vi "CSM-FileSync.vi"(5 "Name(FileSync)":string="FileSync", 7 "Protocol.lvclass":refnum<class "Protocol.lvclass">, 8 "error in":errorcluster, 11 "FileSync Configuration":T1={"MonitoringFolder"=path "_sync/Monitoring", "BackupFolder"=path "_sync/backup", "autostart"=TRUE, "Backup"=FALSE}) -> (0 "error out":errorcluster)   [LabVIEW 2020, in "CSM-FileSync.lvlib"]
doc: "------------- lvcsm -------------\n[CSMStates]\nItem 0 = \"Idle\"\nItem 1 = \"Timeout\"\nItem 2 = \"Initialize Core Data\"\nItem 3 = \"Error Handler\"\nItem 4 = \"VI Reference\"\nItem 5 = \"Exit\"\nItem 6 = \"Data: Initialize\"\nItem 7 = \"Data: Load Configuration\"\nItem 8 = \"Data: Save Configuration\"\nItem 9 = \"Data: Cleanup\"\nItem 10 = \"UI: Initialize\"\nItem 11 = \"UI: Cursor Set\"\nItem 12 = \"UI: Front Panel State\"\nItem 13 = \"UI: Publish Status\"\nItem 14 = \"Macro: Initialize\"\nItem 15 = \"Macro: FileSync Protocol Connect\"\nItem 16 = \"Macro: Check Is Still Alive\"\nItem 17 = \"Macro: FileSync Routines\"\nItem 18 = \"Macro: FileSync Protocol Disconnect\"\nItem 19 = \"Macro: Exit\"\nItem 20 = \"API: Start\"\nItem 21 = \"API: Stop\"\nItem 22 = \"FileSync: Load Configuration\"\nItem 23 = \"FileSync: Try to Connect\"\nItem 24 = \"FileSync: Status Check\"\nItem 25 = \"FileSync: Close Connection\"\nItem 26 = \"FileSync: Cleanup Protocol\"\nItem 27 = \"FileSyncRountine: Create Dir if Not Exist\"\nItem 28 = \"FileSyncRountine: List Files\"\nItem 29 = \"FileSyncRountine: Pick Uploading File\"\nItem 30 = \"FileSyncRountine: Upload\"\nItem 31 = \"FileSyncRountine: Move File to Backup Folder\"\nItem 32 = \"FileSyncRountine: Remove Empty Container Folder\"\n\n[CSMStatus]\nItem 0 = \"Status Change@UI: Publish Status\"\nItem 1 = \"Uploading List Change@UI: Publish Status\""
uses:
  CSM-FileSync.lvlib
  _fileSync_Support/Base/Protocol/Protocol.lvclass
  _fileSync_Support/Base/Def-FileSyncConfig.ctl
  c11ad69d-c218-40bd-9883-d3361c9d07ec.vi
  4f3a877e-8c3a-40cf-89f4-fda6eeae6ffa.vi
  d714c97a-ade9-4c5a-b010-05319b638c8a.vi
  16b40464-5854-4f01-88e3-2a837e9228b3.vi
  16b40464-5854-4f01-88e3-2a837e9228b3.vi/eb2405bd-5b2e-436b-9bb3-692ecf4a9268.vi
  16b40464-5854-4f01-88e3-2a837e9228b3.vi/c8ad12e3-5e6d-40e1-92e0-1426ef45ec41.vi
  16b40464-5854-4f01-88e3-2a837e9228b3.vi/effcbc1a-e97c-42d4-b61f-d821de102707.vi
  <userlib>/_NEVSTOP/Communicable State Machine(CSM)/addons/MassData-Parameter/_support/FGV-MassData(lvlibp).vi
  <userlib>/_NEVSTOP/Communicable State Machine(CSM)/_Polymophic/Add State(s) to Queue By BOOL(Element).vi
  <userlib>/_NEVSTOP/Communicable State Machine(CSM)/_Polymophic/Build Status Broadcast Message.vi
  <userlib>/_NEVSTOP/Communicable State Machine(CSM)/AdvanceAPI/CSM - Set Module Attribute.vi
  <userlib>/_NEVSTOP/Communicable State Machine(CSM)/addons/API-String-Arugments-Support/_Support/Data To API String Arguments.vi
  <userlib>/_NEVSTOP/Communicable State Machine(CSM)/Communicable State Machine.lvlib
  <userlib>/_NEVSTOP/Communicable State Machine(CSM)/addons/Logger/CSM File Logger.lvlib
  <userlib>/_NEVSTOP/Communicable State Machine(CSM)/addons/Loop-Support/CSM Loop Support.lvlib
  <userlib>/_NEVSTOP/Communicable State Machine(CSM)/addons/MassData-Parameter/CSM MassData Parameter Support.lvlib
panel:
  out "State History":string
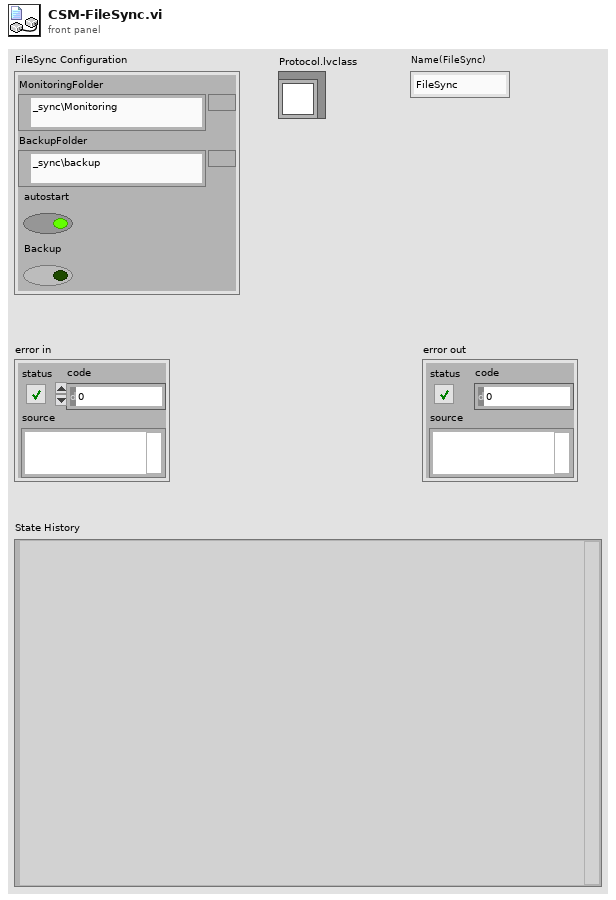
[diagram p1: front panel]
types:
  T1 = typedef "FileSync -- Base.lvlib/Protocol.lvclass/Def-FileSyncConfig.ctl" = cluster{"MonitoringFolder":path, "BackupFolder":path, "autostart":bool, "Backup":bool}
  T2 = enum32{"Invalid", "Standard", "Closed", "Hidden", "Minimized", "Maximized"}
  T3 = enum32{"invalid app kind", "Development System", "Run Time System", "Student Edition", "Embedded LabVIEW", "Evaluation", "Custom"}
  T4 = cluster{"Upload List":path[], "UploadingFile":path}
  T5 = typedef "Communicable State Machine.lvlib/_CSM_Response Source Message.ctl" = cluster{"‘State":string, "’Arguments":string, "’Error":errorcluster}
  T6 = cluster{"Core":cluster{"Current VI Reference":refnum<vi>, "Close Panel on Exit?":bool}, "Configuration":T1, "FileSync Status":cluster{"Connected":bool}, "Upload List":path[], "Temp:UploadingFile":path}
  T7 = cluster{"Current VI Reference":refnum<vi>, "Close Panel on Exit?":bool}
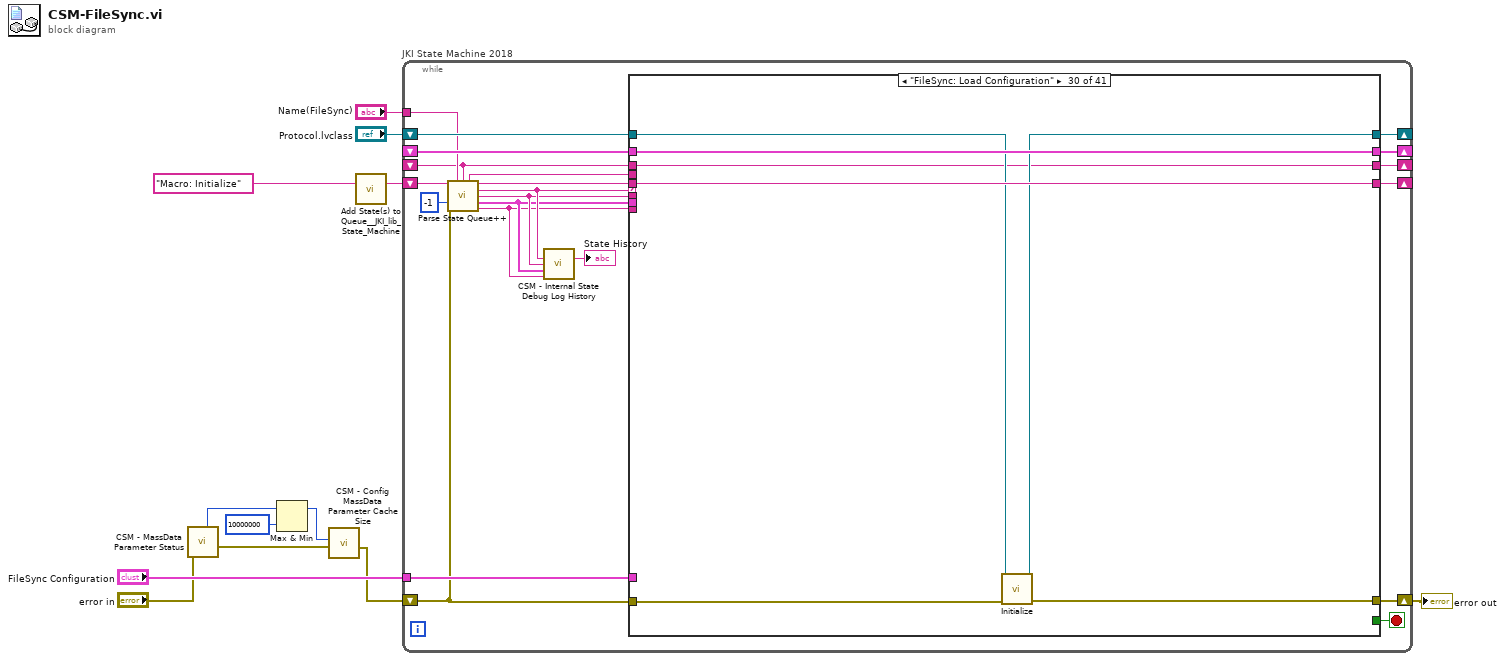
[diagram p0: block diagram]
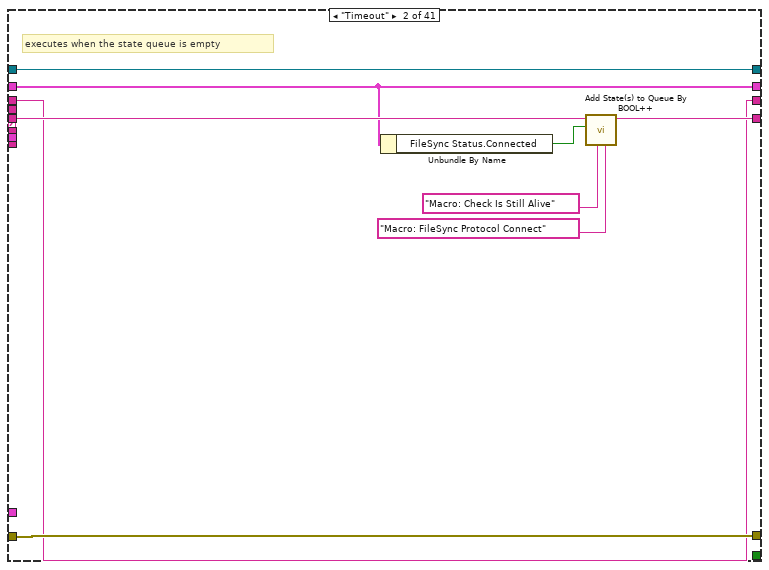
[diagram p3: hidden frame]
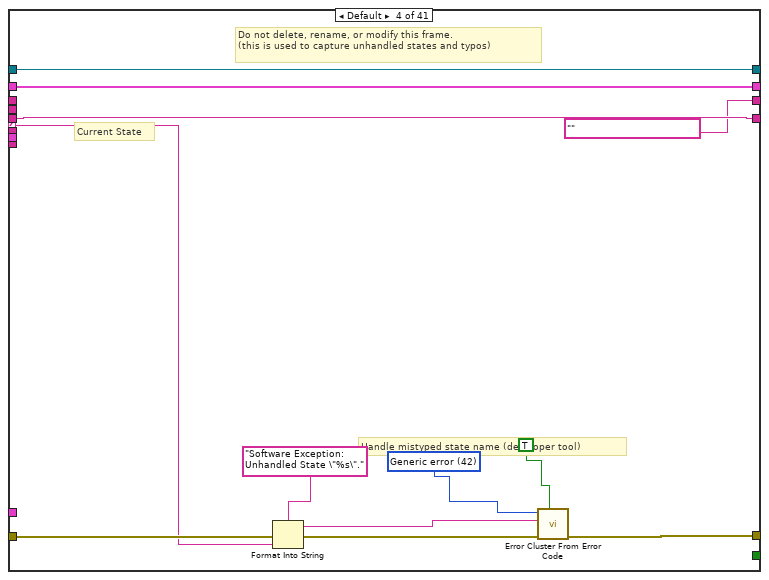
[diagram p5: hidden frame]
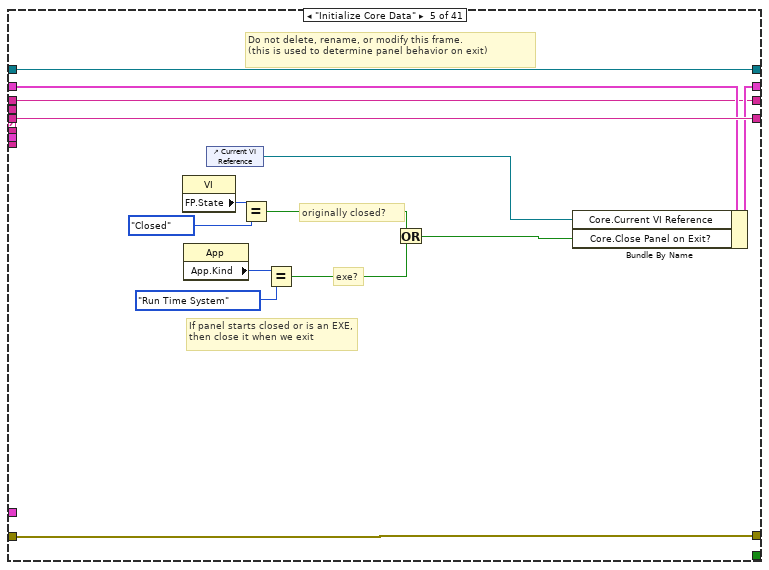
[diagram p6: hidden frame]
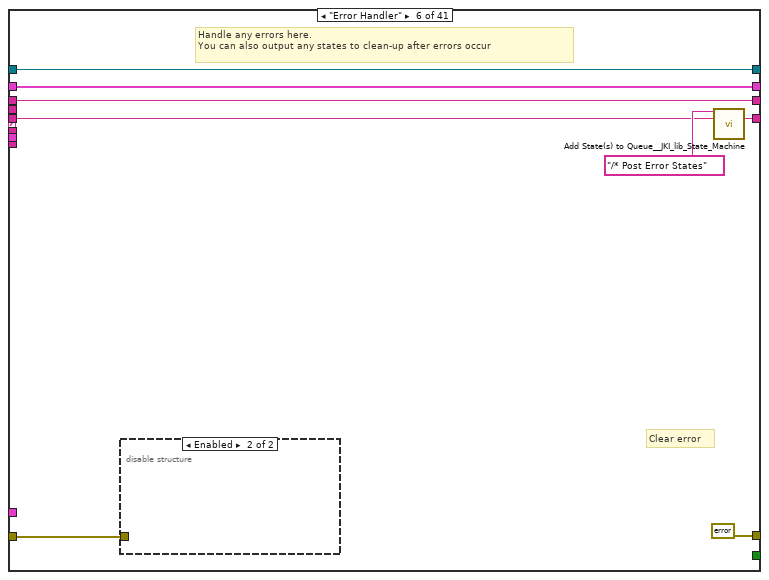
[diagram p7: hidden frame]
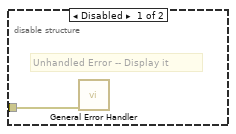
[diagram p8: hidden frame]
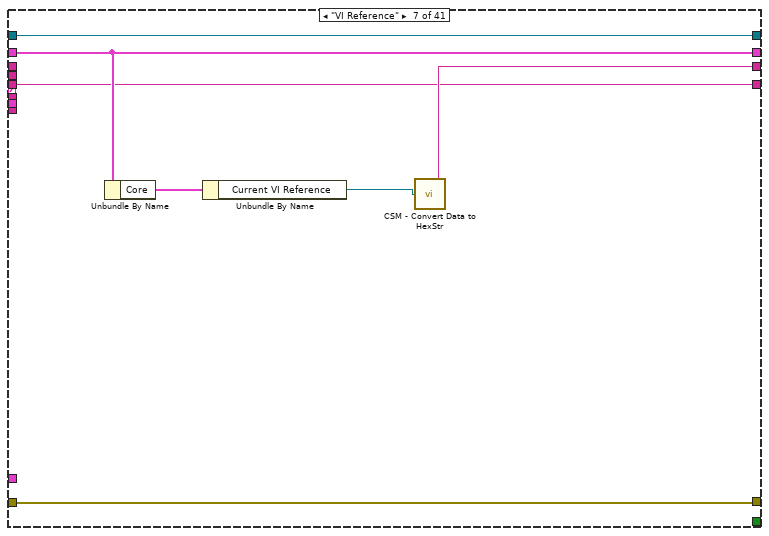
[diagram p9: hidden frame]
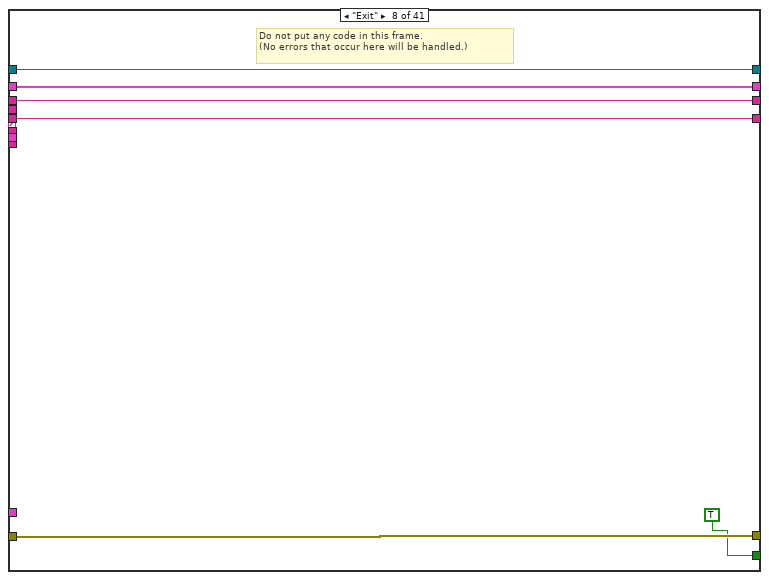
[diagram p10: hidden frame]
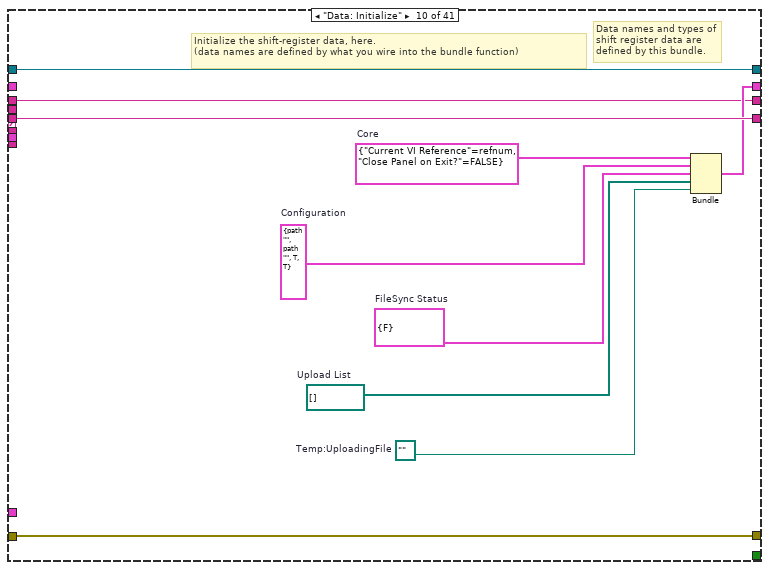
[diagram p12: hidden frame]
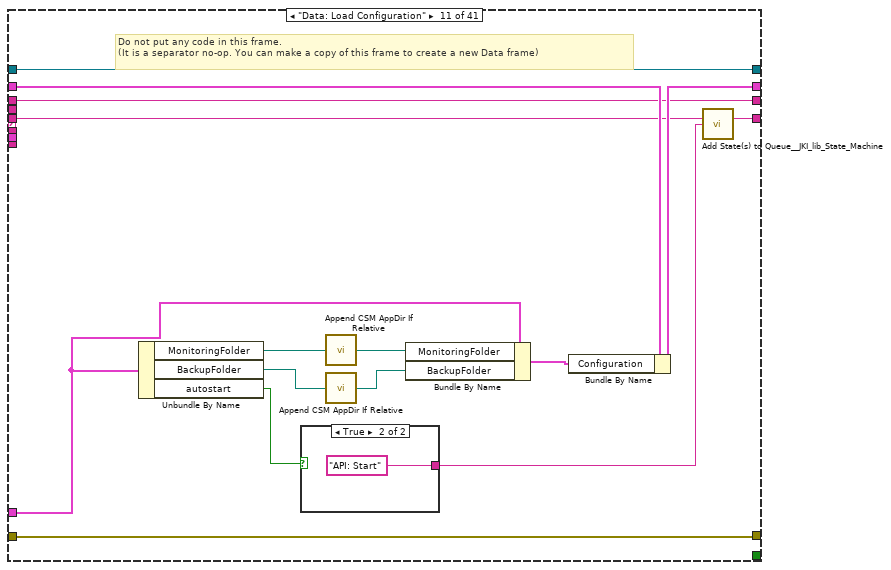
[diagram p13: hidden frame]
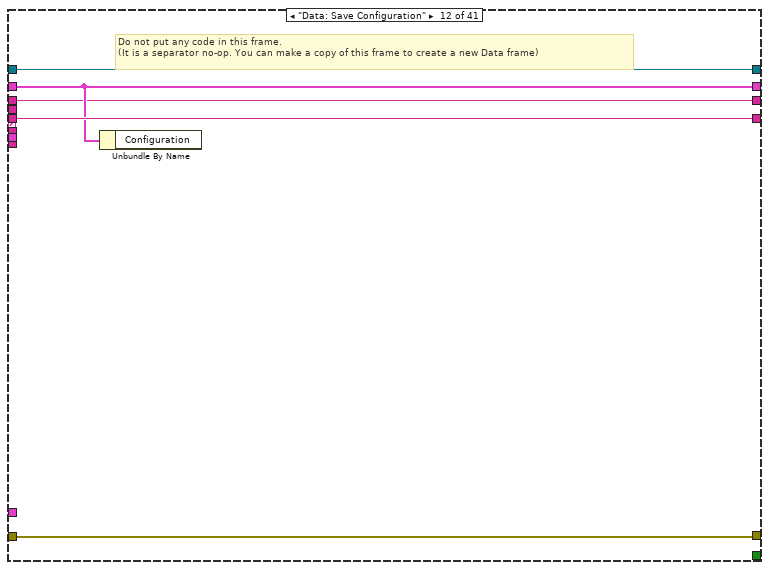
[diagram p15: hidden frame]
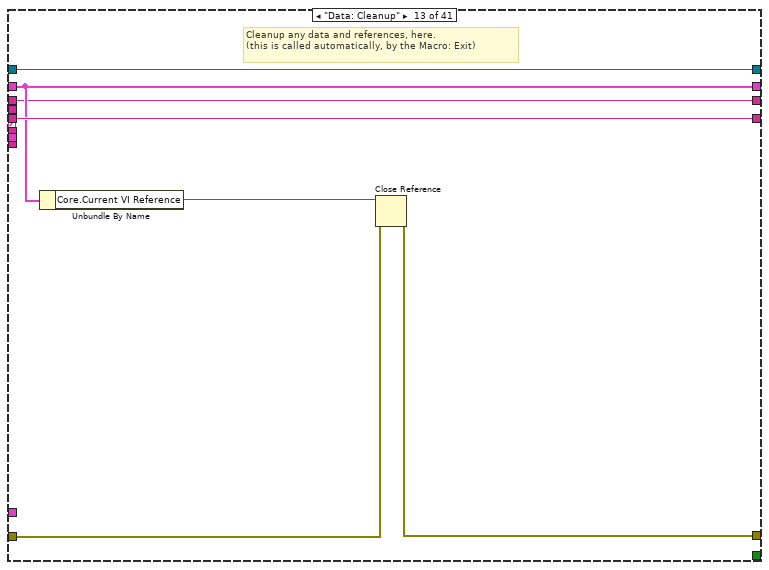
[diagram p16: hidden frame]
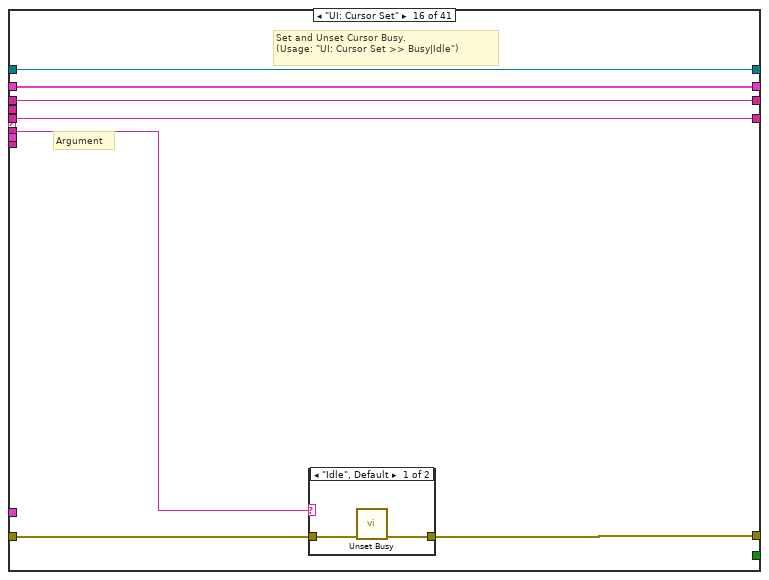
[diagram p19: hidden frame]
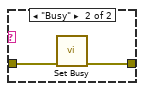
[diagram p20: hidden frame]
diagram:
  n1 = call <userlib>:"CSM - MassData Parameter Status.vi"("Error in"="error in") -> ("Error out"=w6:errorcluster, "Cache Size"=w2:i32)  [unwired: 6 in, 2 out]
  n2 = Max & Min(x=w2, y=10000000) -> (max(x,y)=w3:i32)  [unwired: 1 out]
  n3 = call <userlib>:"CSM - Config MassData Parameter Cache Size.vi"("Error in"=w6, "Size (50M)"=w3) -> ("Error out"=w5:errorcluster)  [unwired: 9 in]
  n4 = call <vilib>:"Add State(s) to Queue__JKI_lib_State_Machine.vi"("State(s) in (\"\")"="Macro: Initialize") -> ("States Out"=w12:string)  [unwired: 14 in]
  n5 = while "JKI State Machine 2018" {
    shift-right: [w30] -> _
    shift-left: _ -> [w29]
    shift-right: [w33] -> w10
    shift-left: w5 -> [w24]
    shift-right: [w32] -> _
    shift-left: w12 -> [w25]
    shift-right: [w27] -> _
    shift-left: "Protocol.lvclass" -> [w28]
    tunnel: "FileSync Configuration" -> [w26]
    shift-right: [w22] -> _
    shift-left: _ -> [w19]
    tunnel: "Name(FileSync)" -> [w21]
    stop <- w31 stop-if-true
    n6 = call <userlib>:"Parse State Queue++.vi"("State Queue"=w25, "Name (\"\" to Use UUID)"=w21, "Response Arguments"=w19, "Previous Error"=w24, "Dequeue (1 ms)"=-1 ("Dequeue Timeout(1ms)")) -> ("Name Used"=w20:string, "Remaining States"=w23:string, "Current State"=w17:string, "Arguments"=w16:string, "Additional Information"=w15:T5, "Source CSM"=w14:string)  [unwired: 5 in]
    n7 = call <userlib>:"CSM - Internal State Debug Log History.vi"("State"=w17, "Arguments (\"\")"=w16, ">> Response Source Message >>"=w15, "Source (\"\")"=w14) -> ("Debug Log"=→"State History":string)  [unwired: 11 in]
    n8 = case shown="\"FileSync: Load Configuration\"" w17 {
      selector: w17 -> [_ _ _ w55 _ _ _ _ _ _ _ _ _ _ _ _ _ _ _ _ _ _ _ _ _ _ _ _ _ _ _ w359 _ _ _ _ _ _ _ _ _]
      tunnel: w23 -> [w34 w47 w52 w58 w78 w79 w90 w100 w105 w115 w119 w136 w143 w148 w153 w160 w172 w250 w262 w269 w274 w282 w293 w302 w318 w321 w327 w332 w338 w345 w354 w360 w377 w384 w389 w397 w406 w422 w432 w458 w500]
      tunnel: w16 -> [_ _ _ _ _ _ _ _ _ _ _ _ _ _ _ w156 w167 _ _ _ _ _ _ _ _ _ _ _ _ _ _ _ _ _ _ _ _ _ w440 w449 w494]
      tunnel: w29 -> [w37 w44 w50 w57 w72 w84 w94 w99 w103 _ w128 w134 w139 w146 w152 w159 w169 w255 w260 w266 w272 w280 w291 w300 w315 w320 w326 w331 w336 w344 w353 w364 w376 w383 w387 w394 w404 w418 w437 w456 w496]
      tunnel: [w38 w45 w51 w60 w76 errorcluster {"status"=FALSE, "code"=0, "source"=""} ("error out") w89 w98 w104 w113 w127 w133 w140 w147 w151 w157 w170 w256 w261 w267 w276 w284 w295 w304 w316 w322 w328 w333 w337 w342 w349 w367 w374 w381 w388 w390 w402 w420 w424 w453 w497] -> w33
      tunnel: w24 -> [w38 w45 w51 w59 w76 w83 w89 w98 w104 w113 w127 w133 w141 w147 w151 w158 w171 w256 w261 w267 w276 w284 w295 w304 w316 w322 w328 w333 w337 w343 w350 w368 w375 w382 w388 _ w401 w420 w438 _ w498]
      tunnel: [w34 w46 w52 w58 w78 w86 w90 w100 w105 w115 w120 w136 w143 w148 w153 w160 w172 w251 w262 w268 w275 w283 w294 w303 w317 w321 w324 w329 w338 w345 w354 w361 w377 w384 w389 w397 w406 w421 w433 w458 w500] -> w32
      tunnel: [_ _ _ _ _ _ _ TRUE _ _ _ _ _ _ _ _ _ _ _ _ _ _ _ _ _ _ _ _ _ _ _ _ _ _ _ _ _ _ _ _ _] -> w31
      tunnel: [w37 w44 w50 w57 w77 w84 w94 w99 w103 w114 w129 w134 w139 w146 w152 w159 w169 w255 w260 w266 w272 w280 w291 w300 w315 w320 w326 w331 w336 w344 w348 w364 w371 w383 w387 w394 w400 w417 w437 w450 w496] -> w30
      tunnel: w28 -> [w36 w43 w49 w54 w66 w81 w88 w96 w102 w111 w130 w135 w138 w145 w150 w155 w166 w257 w259 w264 w277 w285 w296 w305 w308 w319 w325 w330 w335 w341 w352 w366 w373 w380 w386 w396 w405 w419 w435 w457 w499]
      tunnel: [w36 w43 w49 w54 w66 w81 w88 w96 w102 w111 w130 w135 w138 w145 w150 w155 w166 w257 w259 w264 w277 w285 w296 w305 w308 w319 w325 w330 w335 w340 w351 w365 w372 w379 w386 w396 w405 w419 w439 w457 w499] -> w27
      tunnel: w26 -> [_ _ _ _ _ _ _ _ _ _ w116 _ _ _ _ _ _ _ _ _ _ _ _ _ _ _ _ _ _ _ _ _ _ _ _ _ _ _ _ _ _]
      tunnel: [w35 w42 w48 "" ("message") w65 w80 w91 w95 w101 w106 w125 w132 w137 w144 w149 w154 w165 w254 w258 w263 w270 w279 w292 w298 w307 _ _ _ w334 w339 w346 w363 w369 w378 w385 w391 w398 w410 w434 w452 w491] -> w22
      tunnel: w14 -> [_ _ _ _ _ _ _ _ _ _ _ _ _ _ _ _ _ _ _ _ _ _ _ _ _ _ _ _ _ _ _ _ _ _ _ _ _ _ _ _ _]
      tunnel: w15 -> [_ _ _ _ _ _ _ _ _ _ _ _ _ _ _ _ _ _ _ _ _ _ _ _ _ _ _ _ _ _ _ _ _ _ _ _ _ _ _ _ _]
      tunnel: w20 -> [_ _ _ _ _ _ _ _ _ _ _ _ _ _ _ _ _ w253 _ _ _ _ _ _ _ _ _ _ _ _ _ _ _ _ _ _ _ _ _ _ _]
      tunnel: w19 -> [w35 w42 w48 _ w65 w80 _ w95 w101 w106 w125 w132 w137 w144 w149 w154 w165 w254 w258 w263 w270 w279 w292 w298 w307 _ _ _ w334 w339 w346 w363 w369 w378 w385 w391 w398 w410 w434 w452 w491]
      frame "", "Idle" {
      }
      frame "Timeout" {
        # "executes when the state queue is empty"
        n9 = Unbundle By Name(w44) -> ("FileSync Status.Connected"=w39:bool)
        n10 = call-poly <userlib>:"Add State(s) to Queue By BOOL++.vi"("FALSE (\"\")"="Macro: FileSync Protocol Connect" ("State(s) in Front (\"\")"), "TRUE (\"\")"="Macro: Check Is Still Alive" ("State(s) in Front (\"\")"), "Condition"=w39, "State Queue (\"\")"=w47) -> ("Remaining States"=w46:string)  [unwired: 7 in]
      }
      frame "---------- Core ----------" {
        # "Do not put any code in this frame.\n(it is a separator no-op)"
      }
      frame Default {
        w63 = 42 items=["No error", "Argument error", "Memory is full", "Out of zone", "End of file", "File already open", "Generic file I/O error", "File not found", "File permission error", "Disk is full", "Duplicate path", "Too many files open", "System feature not enabled", "Resource file not found", "Cannot add resource", "Resource not found", "Image not found", "Image memory error", "Pen does not exist", "Config type invalid", "Config token not found", "Config parse error", "Config memory error", "Bad external code format", "Bad external code offset", "External code not present", "Null window", "Destroy window error", "Null menu", "Print aborted", "Bad print record", "Print driver error", "Windows error during printing", "Memory error during printing", "Print dialog error", "Generic print error", "Invalid device refnum", "Device not found", "Device parameter error", "Device unit error", "Cannot open device", "Device call aborted", "Generic error", "Cancelled by user", "Object ID too low", "Object ID too high", "Object not in heap", "Unknown heap", "Unknown object (invalid DefProc)", "Unknown object (DefProc not in table)", "Message out of range", "Invalid (null) method", "Unknown message", "Manager call not supported", "Bad address", "Network operation in progress", "Network operation timed out", "Connection is busy", "Network attribute not supported", "Network error", "Address in use", "System out of memory", "Connection aborted", "Connection refused", "Not connected", "Already connected", "Connection closed", "Initialization error (interapplication manager)", "Bad occurrence", "Wait on unbound occurrence handler", "Occurrence queue overflow", "Datalog type conflict", "Unused", "Unrecognized type (interapplication manager)", "Memory corrupt", "Failed to make temporary DLL", "Old CIN version", "Drag socket not found", "Failed to load drop-object", "Failed to register OLE object", "Failed to release OLE object", "Format specifier type mismatch", "Unknown format specifier", "Too few format specifiers", "Too many format specifiers", "Scan failed", "Newer CIN version", "Error converting to variant", "Runtime menu error", "Password tampered", "Variant attribute not found", "Incompatible variant data type", "Event data is not available", "Event Store is not present", "Occurrence is not found", "Event Queue is not created", "Event info is not available", "Refnum passed is NULL", "Error retrieving Class GUID", "Error retrieving CoClass GUID", "Error retrieving TypeLib GUID.", "Bad built application magic bytes.", "Specific driver is different from the specific driver associated with the Logical Name.", "There is no session opened to the class driver.", "Max Error", "MAX - Error with config objects", "MAX - Error loading configuration", "MAX - Group not supported"]
        # "Current State"
        # "Do not delete, rename, or modify this frame.\n(this is used to capture unhandled states and typos)"
        # "Handle mistyped state name (developer tool)"
        n11 = Format Into String(format string="Software Exception: Unhandled State \"%s\"." ("message"), error in=w59, w55) -> (resulting string=w62:string, error out=w61:errorcluster)  [unwired: 1 in]
        n12 = call <vilib>:"Error Cluster From Error Code.vi"("show call chain? (False)"=TRUE, "error in (no error)"=w61, "error message (\"\")"=w62, "error code (0)"=w63) -> ("error out"=w60:errorcluster)  [unwired: 5 in]
      }
      frame "Initialize Core Data" {
        # "Do not delete, rename, or modify this frame.\n(this is used to determine panel behavior on exit)"
        # "originally closed?"
        # "exe?"
        # "If panel starts closed or is an EXE, then close it when we exit"
        n13 = property class="VI"() -> ("FP.State"=w69:T2)  [unwired: 2 in, 2 out]
        n14 = property class="App"() -> ("App.Kind"=w75:T3)  [unwired: 2 in, 2 out]
        n15 = control-ref of="Current VI Reference"() -> (w70:refnum<vi>)
        n16 = Equal?(x=w69, y=T2."Closed" ("Front Panel Window:State")) -> (x = y?=w67:bool)
        n17 = Equal?(x=w75, y=T3."Run Time System" ("Application:Kind")) -> (x = y?=w73:bool)
        n18 = Or(x=w67, y=w73) -> (x .or. y?=w71:bool)
        n19 = Bundle By Name(cluster=w72, "Core.Current VI Reference"=w70, "Core.Close Panel on Exit?"=w71) -> (w77:T6)
      }
      frame "Error Handler" {
        # "Handle any errors here.\nYou can also output any states to clean-up after errors occur"
        # "Clear error"
        n20 = disable-structure shown="Enabled" {
          disable-tunnel: w83 -> [w87 _]
          frame Disabled {
            # "Unhandled Error -- Display it"
            n21 = call <vilib>:"General Error Handler.vi"("error in (no error)"=w87) -> ()  [unwired: 10 in, 5 out]
          }
          frame Enabled {
          }
        }
        n22 = call <vilib>:"Add State(s) to Queue__JKI_lib_State_Machine.vi"("State(s) in Front (\"\")"="/* Post Error States", "State(s) in (\"\")"=w79) -> ("States Out"=w86:string)  [unwired: 13 in]
      }
      frame "VI Reference" {
        n23 = Unbundle By Name(w94) -> ("Core"=w93:T7)
        n24 = Unbundle By Name(w93) -> ("Current VI Reference"=w92:refnum<vi>)
        n25 = call <userlib>:"CSM - Convert Data to HexStr.vi"("Variant"=w92) -> ("HEX String (0-9,A-F)"=w91:string)  [unwired: 8 in]
      }
      frame "Exit" {
        # "Do not put any code in this frame.\n(No errors that occur here will be handled.)"
      }
      frame "---------- Data ----------" {
        # "Do not put any code in this frame.\n(It is a separator no-op. You can make a copy of this frame to create a new Data frame)"
      }
      frame "Data: Initialize" {
        w107 = path ""  # Temp:UploadingFile
        w108 = path[] []  # Upload List
        w109 = cluster{"Connected":bool} {"Connected"=FALSE}  # FileSync Status
        w110 = T1 {"MonitoringFolder"=path "", "BackupFolder"=path "", "autostart"=TRUE, "Backup"=TRUE}  # Configuration
        w112 = T7 {"Current VI Reference"=refnum, "Close Panel on Exit?"=FALSE}  # Core
        # "Data names and types of shift register data are defined by this bundle."
        # "Initialize the shift-register data, here.\n(data names are defined by what you wire into the bundle function)"
        n26 = Bundle("Core"=w112, "Configuration"=w110, "FileSync Status"=w109, "Upload List"=w108, "Temp:UploadingFile"=w107) -> (w114:T6)  [unwired: 1 in]
      }
      frame "Data: Load Configuration" {
        # "Do not put any code in this frame.\n(It is a separator no-op. You can make a copy of this frame to create a new Data frame)"
        n27 = Unbundle By Name(w116) -> ("MonitoringFolder"=w124:path, "BackupFolder"=w123:path, "autostart"=w117:bool)
        n28 = case shown="True" w117 {
          tunnel: [_ "API: Start" ("State(s) at Back (\"\")")] -> w118
          frame False {
          }
          frame True {
          }
        }
        n29 = call <userlib>:"Append CSM AppDir If Relative.vi"("Relative Path (.)"=w124) -> ("Application Directory (+ Relative)"=w122:path)  [unwired: 4 in]
        n30 = call <userlib>:"Append CSM AppDir If Relative.vi"("Relative Path (.)"=w123) -> ("Application Directory (+ Relative)"=w121:path)  [unwired: 4 in]
        n31 = Bundle By Name(cluster=w116, "MonitoringFolder"=w122, "BackupFolder"=w121) -> (w126:T1)
        n32 = Bundle By Name(cluster=w128, "Configuration"=w126) -> (w129:T6)
        n33 = call <vilib>:"Add State(s) to Queue__JKI_lib_State_Machine.vi"("State(s) in (\"\")"=w119, "State(s) at Back (\"\")"=w118) -> ("States Out"=w120:string)  [unwired: 13 in]
      }
      frame "Data: Save Configuration" {
        # "Do not put any code in this frame.\n(It is a separator no-op. You can make a copy of this frame to create a new Data frame)"
        n34 = Unbundle By Name(w134) -> ()  [unwired: 1 out]
      }
      frame "Data: Cleanup" {
        # "Cleanup any data and references, here.\n(this is called automatically, by the Macro: Exit)"
        n35 = Unbundle By Name(w139) -> ("Core.Current VI Reference"=w142:refnum<vi>)
        n36 = Close Reference(reference=w142, error in (no error)=w141) -> (error out=w140:errorcluster)
      }
      frame "---------- UI ----------" {
        # "Do not put any code in this frame.\n(It is a separator no-op. You can make a copy of this frame to create a new UI frame)"
      }
      frame "UI: Initialize" {
      }
      frame "UI: Cursor Set" {
        # "Argument"
        # "Set and Unset Cursor Busy.\n(Usage: \"UI: Cursor Set >> Busy|Idle\")"
        n37 = case shown="\"Idle\", Default" w156 {
          tunnel: w158 -> [w162 w164]
          tunnel: [w161 w163] -> w157
          frame "Idle", Default {
            n38 = call <vilib>:"Unset Busy.vi"("error in (no error)"=w162) -> ("error out"=w161:errorcluster)  [unwired: 10 in]
          }
          frame "Busy" {
            n39 = call <vilib>:"Set Busy.vi"("error in (no error)"=w164) -> ("error out"=w163:errorcluster)  [unwired: 9 in, 1 out]
          }
        }
      }
      frame "UI: Front Panel State" {
        # "Argument"
        # "Set Front Panel Open or Closed\n(Usage: \"UI: Front Panel State >> Open|Close\")"
        n40 = Unbundle By Name(w169) -> ("Core.Current VI Reference"=w168:refnum<vi>)
        n41 = case shown="\"Open\", \"Standard\", Default" w167 {
          tunnel: w171 -> [w178 w193 w204 w217 w230]
          tunnel: [w180 w194 w206 w219 w232] -> w170
          tunnel: w168 -> [w179 w191 w205 w218 w231]
          frame "Open", "Standard", Default {
            w173 = T2."Standard" ("State")
            n42 = property class="VI"(reference=w179, error in=w178) -> (reference out=w176:refnum<vi>, error out=w177:errorcluster, "FP.State"=w175:T2)
            n43 = Not Equal?(x=w175, y=w173) -> (x != y?=w174:bool)
            n44 = case shown="True" w174 {
              tunnel: [w184 w186] -> w180
              tunnel: w177 -> [w183 w186]
              tunnel: w176 -> [w182 _]
              tunnel: w173 -> [w181 _]
              frame True {
                n45 = invoke class="VI" method="FP.Open"(reference=w182, error in=w183, "Activate"=TRUE, "State"=w181) -> (error out=w184:errorcluster)  [unwired: 1 in, 4 out]
              }
              frame False {
              }
            }
          }
          frame "Close", "Closed" {
            n46 = property class="VI"(reference=w191, error in=w193) -> (reference out=w190:refnum<vi>, error out=w192:errorcluster, "FP.State"=w188:T2)
            n47 = Not Equal?(x=w188, y=T2."Closed" ("Front Panel Window:State")) -> (x != y?=w187:bool)
            n48 = case shown="True" w187 {
              tunnel: [w195 w198] -> w194
              tunnel: w192 -> [w195 w197]
              tunnel: w190 -> [_ w196]
              frame False {
              }
              frame True {
                n49 = invoke class="VI" method="FP.Close"(reference=w196, error in=w197) -> (error out=w198:errorcluster)  [unwired: 1 in, 2 out]
              }
            }
          }
          frame "Hidden", "Hide" {
            w199 = T2."Hidden" ("State")
            n50 = property class="VI"(reference=w205, error in=w204) -> (reference out=w202:refnum<vi>, error out=w203:errorcluster, "FP.State"=w201:T2)
            n51 = Not Equal?(x=w201, y=w199) -> (x != y?=w200:bool)
            n52 = case shown="True" w200 {
              tunnel: [w210 w211] -> w206
              tunnel: w203 -> [w209 w211]
              tunnel: w202 -> [w208 _]
              tunnel: w199 -> [w207 _]
              frame True {
                n53 = invoke class="VI" method="FP.Open"(reference=w208, error in=w209, "State"=w207) -> (error out=w210:errorcluster)  [unwired: 2 in, 4 out]
              }
              frame False {
              }
            }
          }
          frame "Minimize", "Minimized" {
            w212 = T2."Minimized" ("State")
            n54 = property class="VI"(reference=w218, error in=w217) -> (reference out=w215:refnum<vi>, error out=w216:errorcluster, "FP.State"=w214:T2)
            n55 = Not Equal?(x=w214, y=w212) -> (x != y?=w213:bool)
            n56 = case shown="True" w213 {
              tunnel: [w223 w224] -> w219
              tunnel: w216 -> [w222 w224]
              tunnel: w215 -> [w221 _]
              tunnel: w212 -> [w220 _]
              frame True {
                n57 = invoke class="VI" method="FP.Open"(reference=w221, error in=w222, "State"=w220) -> (error out=w223:errorcluster)  [unwired: 2 in, 4 out]
              }
              frame False {
              }
            }
          }
          frame "Maximize", "Maximized" {
            w225 = T2."Maximized" ("State")
            n58 = property class="VI"(reference=w231, error in=w230) -> (reference out=w228:refnum<vi>, error out=w229:errorcluster, "FP.State"=w227:T2)
            n59 = Not Equal?(x=w227, y=w225) -> (x != y?=w226:bool)
            n60 = case shown="True" w226 {
              tunnel: [w236 w237] -> w232
              tunnel: w229 -> [w235 w237]
              tunnel: w228 -> [w234 _]
              tunnel: w225 -> [w233 _]
              frame True {
                n61 = invoke class="VI" method="FP.Open"(reference=w234, error in=w235, "State"=w233) -> (error out=w236:errorcluster)  [unwired: 2 in, 4 out]
              }
              frame False {
              }
            }
          }
        }
      }
      frame "UI: Publish Status" {
        n62 = Unbundle By Name(w255) -> ("FileSync Status.Connected"=w249:bool, "Upload List"=w238:path[], "Temp:UploadingFile"=w248:path)
        n63 = call "CSM Set Module Attribute.vim"("CSM Name"=w253, "Attribute"="Connected", "Value"=w249) -> ()  [unwired: 9 in, 4 out]
        n64 = Bundle(cluster=T4 {"Upload List"=[], "UploadingFile"=path ""} ("output cluster"), "Upload List"=w238, "UploadingFile"=w248) -> (w246:T4)
        n65 = call "Convert Data To API String Arguments.vim"("Data"=w249) -> ("API String"=w239:string)  [unwired: 7 in, 1 out]
        n66 = call "CSM - Convert MassData to Argument.vim"("Data"=w246) -> ("MassData Argument"=w241:string)  [unwired: 7 in, 1 out]
        n67 = call-poly <userlib>:"Build Message with Arguments++.vi"("State With Arguments"="Status Change" ("Attribute"), "Arguments (\"\")"=w239) -> ("CSM Message String"=w245:string)  [unwired: 13 in]
        n68 = call-poly <userlib>:"Build Message with Arguments++.vi"("State With Arguments"="Uploading List Change" ("Attribute"), "Arguments (\"\")"=w241) -> ("CSM Message String"=w244:string)  [unwired: 13 in]
        n69 = call <vilib>:"Add State(s) to Queue__JKI_lib_State_Machine.vi"("State(s) in (\"\")"=w245, "State(s) at Back (\"\")"=w244) -> ("States Out"=w243:string)  [unwired: 13 in]
        n70 = call <vilib>:"Add State(s) to Queue__JKI_lib_State_Machine.vi"("State(s) in Front (\"\")"=w243, "State(s) in (\"\")"=w250) -> ("States Out"=w251:string)  [unwired: 13 in]
      }
      frame "---------- Macro ----------" {
        # "Do not put any code in this frame.\n(It is a separator no-op. You can make a copy of this frame to create a new Macro frame)"
      }
      frame "Macro: Initialize" {
        # "Initialization Macro\n(This is called once, when the VI starts)"
        n71 = call <vilib>:"Add State(s) to Queue__JKI_lib_State_Machine.vi"("State(s) in Front (\"\")"="Data: Initialize\nInitialize Core Data\nData: Load Configuration\nUI: Initialize\nUI: Publish Status\n//UI: Front Panel State >> Open\n", "State(s) in (\"\")"=w269) -> ("States Out"=w268:string)  [unwired: 13 in]
      }
      frame "Macro: FileSync Protocol Connect" {
        n72 = Unbundle By Name(w272) -> ("FileSync Status.Connected"=w271:bool)
        n73 = case shown="True" w271 {
          tunnel: [_ "FileSync: Load Configuration\nFileSync: Try to Connect\nUI: Publish Status" ("State(s) in Front (\"\")")] -> w273
          frame False {
          }
          frame True {
          }
        }
        n74 = call <vilib>:"Add State(s) to Queue__JKI_lib_State_Machine.vi"("State(s) in Front (\"\")"=w273, "State(s) in (\"\")"=w274) -> ("States Out"=w275:string)  [unwired: 13 in]
      }
      frame "Macro: Check Is Still Alive" {
        n75 = call <vilib>:"Add State(s) to Queue__JKI_lib_State_Machine.vi"("State(s) in Front (\"\")"="FileSync: Check Connection is Still Alive" ("State(s) in Front (\"\")"), "State(s) in (\"\")"=w282) -> ("States Out"=w283:string)  [unwired: 13 in]
      }
      frame "Macro: FileSync Routines" {
        n76 = Unbundle By Name(w291) -> ("Upload List"=w290:path[])
        n77 = Empty Array?(array=w290) -> (empty?=w286:bool)
        n78 = case shown="True" w286 {
          tunnel: [_ "FileSyncRountine: Create Dir if Not Exist\nFileSyncRountine: List Files" ("State(s) in Front (\"\")")] -> w289
          frame False {
          }
          frame True {
          }
        }
        n79 = call <vilib>:"Add State(s) to Queue__JKI_lib_State_Machine.vi"("State(s) in Front (\"\")"=w289, "State(s) in (\"\")"="FileSyncRountine: Pick Uploading File\n" ("State(s) in Front (\"\")")) -> ("States Out"=w287:string)  [unwired: 13 in]
        n80 = call <vilib>:"Add State(s) to Queue__JKI_lib_State_Machine.vi"("State(s) in Front (\"\")"=w287, "State(s) in (\"\")"=w293) -> ("States Out"=w294:string)  [unwired: 13 in]
      }
      frame "Macro: FileSync Protocol Disconnect" {
        n81 = Unbundle By Name(w300) -> ("FileSync Status.Connected"=w299:bool)
        n82 = case shown="True" w299 {
          tunnel: [_ "FileSync: Close Connection\nFileSync: Cleanup Protocol\nUI: Publish Status" ("State(s) in Front (\"\")")] -> w301
          frame False {
          }
          frame True {
          }
        }
        n83 = call <vilib>:"Add State(s) to Queue__JKI_lib_State_Machine.vi"("State(s) in Front (\"\")"=w301, "State(s) in (\"\")"=w302) -> ("States Out"=w303:string)  [unwired: 13 in]
      }
      frame "Macro: Exit" {
        # "Exit Macro\n(This is called once, when the VI exits)"
        n84 = Unbundle By Name(w315) -> ("Core.Close Panel on Exit?"=w314:bool)
        n85 = Select(t="//UI: Front Panel State >> Close", s=w314, f="") -> (s? t:f=w311:string)
        n86 = call <vilib>:"Add State(s) to Queue__JKI_lib_State_Machine.vi"("State(s) in (\"\")"=w311, "State(s) at Back (\"\")"="Macro: FileSync Protocol Disconnect\nData: Cleanup\nExit") -> ("States Out"=w309:string)  [unwired: 13 in]
        n87 = call <vilib>:"Add State(s) to Queue__JKI_lib_State_Machine.vi"("State(s) in Front (\"\")"=w309, "State(s) in (\"\")"=w318) -> ("States Out"=w317:string)  [unwired: 13 in]
      }
      frame "---------- API ----------" {
      }
      frame "API: Start" {
        n88 = call <userlib>:"CSMLS - Define Loop State(s).vi"("Loop States"="FileSync: Load Configuration\nFileSync: Try to Connect\nFileSync: Status Check -><loop>\nFileSync: Close Connection\nFileSync: Cleanup Protocol" ("Loop State(s) and Arguments"), "States Queue"=w327) -> ("Remaining States"=w324:string)  [unwired: 13 in]
      }
      frame "API: Stop" {
        n89 = call <userlib>:"CSMLS - Remove Loop Tag and previous State(s) to Break.vi"("States Queue"=w332) -> ("Remaining States"=w329:string)  [unwired: 10 in]
      }
      frame "---------- FileSync ----------" {
      }
      frame "FileSync: Load Configuration" {
        n90 = call-dynamic "Initialize.vi"("error in (no error)"=w343, "Protocol in"=w341) -> ("error out"=w342:errorcluster, "Protocol out"=w340:refnum<class "Protocol.lvclass">)  [unwired: 8 in]
      }
      frame "FileSync: Try to Connect" {
        n91 = call-dynamic "Connect.vi"("error in (no error)"=w350, "Protocol in"=w352) -> ("error out"=w349:errorcluster, "Connected?"=w347:bool, "Protocol out"=w351:refnum<class "Protocol.lvclass">)  [unwired: 7 in]
        n92 = Bundle By Name(cluster=w353, "FileSync Status.Connected"=w347) -> (w348:T6)
      }
      frame "FileSync: Status Check" {
        n93 = call-dynamic "Check.vi"("error in (no error)"=w368, "Protocol in"=w366) -> ("error out"=w367:errorcluster, "Still alive?"=w362:bool, "Protocol out"=w365:refnum<class "Protocol.lvclass">)  [unwired: 7 in]
        n94 = Wait (ms)(milliseconds to wait=u32 200) -> ()  [unwired: 1 out]
        n95 = Select(t="Macro: FileSync Routines" ("State(s) in Front (\"\")"), s=w362, f="Macro: FileSync Protocol Disconnect\nFileSync: Load Configuration\nFileSync: Try to Connect" ("State(s) in Front (\"\")")) -> (s? t:f=w357:string)
        n96 = call <userlib>:"CSMLS - Append Continuous State.vi"("Loop State(s) And Arguments"=w357, "Continous State"=w359, "States Queue"=w360) -> ("Remaining States"=w361:string)  [unwired: 8 in]
      }
      frame "FileSync: Close Connection" {
        n97 = call-dynamic "Disconnect.vi"("error in (no error)"=w375, "Protocol in"=w373) -> ("error out"=w374:errorcluster, "Protocol out"=w372:refnum<class "Protocol.lvclass">)  [unwired: 8 in]
        n98 = Bundle By Name(cluster=w376, "FileSync Status.Connected"=FALSE) -> (w371:T6)
      }
      frame "FileSync: Cleanup Protocol" {
        n99 = call-dynamic "Cleanup.vi"("error in (no error)"=w382, "Protocol in"=w380) -> ("error out"=w381:errorcluster, "Protocol out"=w379:refnum<class "Protocol.lvclass">)  [unwired: 8 in]
      }
      frame "---------- FileSyncRountine ----------" {
      }
      frame "FileSyncRountine: Create Dir if Not Exist" {
        n100 = Unbundle By Name(w394) -> ("Configuration.MonitoringFolder"=w393:path, "Configuration.BackupFolder"=w392:path)
        n101 = call <vilib>:"Create Directory Recursive.vi"("directory"=w393) -> ("error out"=w395:errorcluster)  [unwired: 4 in, 2 out]
        n102 = call <vilib>:"Create Directory Recursive.vi"("error in (no error)"=w395, "directory"=w392) -> ("error out"=w390:errorcluster)  [unwired: 3 in, 2 out]
      }
      frame "FileSyncRountine: List Files" {
        n103 = Unbundle By Name(w404) -> ("Configuration.MonitoringFolder"=w403:path)
        n104 = call <vilib>:"Recursive File List.vi"("error in (no error)"=w401, "Folder Path"=w403) -> ("error out"=w402:errorcluster, "All Files in Dir"=w399:path[])  [unwired: 5 in, 3 out]
        n105 = Bundle By Name(cluster=w404, "Upload List"=w399) -> (w400:T6)
      }
      frame "FileSyncRountine: Pick Uploading File" {
        n106 = Unbundle By Name(w418) -> ("Upload List"=w412:path[])
        n107 = Index Array(array=w412) -> (element=w411:path)  [unwired: 1 in]
        n108 = Path To String(path=w411) -> (string=w413:string)
        n109 = Bundle By Name(cluster=w418, "Temp:UploadingFile"=w411) -> (w417:T6)
        n110 = Empty String/Path?(string/path=w411) -> (empty?=w416:bool)
        n111 = call <vilib>:"Build State String with Arguments__JKI_lib_State_Machine.vi"("Arguments (\"\")"=w413, "State"="FileSyncRountine: Upload" ("False(Empty)")) -> ("State with Arguments"=w408:string)  [unwired: 4 in]
        n112 = call <vilib>:"Add State(s) to Queue__JKI_lib_State_Machine.vi"("State(s) in Front (\"\")"="UI: Publish Status" ("False(Empty)"), "State(s) in (\"\")"=w408) -> ("States Out"=w415:string)  [unwired: 13 in]
        n113 = call-poly <userlib>:"Add State(s) to Queue By BOOL++.vi"("FALSE (\"\")"=w415, "High Priority? (F)"=TRUE ("High Priority(FALSE)"), "Condition"=w416, "State Queue (\"\")"=w422) -> ("Remaining States"=w421:string)  [unwired: 7 in]
      }
      frame "FileSyncRountine: Upload" {
        n114 = String To Path(string=w440) -> (path=w425:path)
        n115 = Unbundle By Name(w437) -> ("Configuration.MonitoringFolder"=w436:path)
        n116 = call-dynamic "UploadFile.vi"("Root Path"=w436, "error in (no error)"=w438, "Path"=w425, "Protocol in"=w435) -> ("error out"=w424:errorcluster, "Protocol out"=w439:refnum<class "Protocol.lvclass">)  [unwired: 6 in]
        n117 = Path To String(path=w425) -> (string=w429:string)
        n118 = call <vilib>:"Build State String with Arguments__JKI_lib_State_Machine.vi"("Arguments (\"\")"=w429, "State"="FileSyncRountine: Move File to Backup Folder" ("False(Empty)")) -> ("State with Arguments"=w430:string)  [unwired: 4 in]
        n119 = call <vilib>:"Build State String with Arguments__JKI_lib_State_Machine.vi"("Arguments (\"\")"=w429, "State"="FileSyncRountine: Remove Empty Container Folder" ("False(Empty)")) -> ("State with Arguments"=w431:string)  [unwired: 4 in]
        n120 = case shown="No Error" w424 {
          tunnel: w431 -> [w442 _]
          tunnel: w430 -> [w443 _]
          tunnel: [w444 _] -> w426
          tunnel: "UI: Publish Status" ("False(Empty)") -> [w441 _]
          frame No Error {
            n121 = call <vilib>:"Add State(s) to Queue__JKI_lib_State_Machine.vi"("State(s) in Front (\"\")"=w443, "State(s) in (\"\")"=w442, "State(s) at Back (\"\")"=w441) -> ("States Out"=w444:string)  [unwired: 12 in]
          }
          frame Error {
          }
        }
        n122 = call <vilib>:"Add State(s) to Queue__JKI_lib_State_Machine.vi"("State(s) in Front (\"\")"=w426, "State(s) in (\"\")"=w432) -> ("States Out"=w433:string)  [unwired: 13 in]
      }
      frame "FileSyncRountine: Move File to Backup Folder" {
        n123 = Unbundle By Name(w456) -> ("Upload List"=w448:path[], "Configuration.Backup"=w451:bool, "Configuration.BackupFolder"=w455:path, "Configuration.MonitoringFolder"=w454:path)
        n124 = String To Path(string=w449) -> (path=w447:path)
        n125 = case shown="True" w451 {
          tunnel: w455 -> [w463 w488]
          tunnel: w454 -> [w462 w487]
          tunnel: [w461 w486] -> w453
          tunnel: w447 -> [w459 w484]
          frame True {
            n126 = Empty String/Path?(string/path=w459) -> (empty?=w460:bool)
            n127 = case shown="False" w460 {
              tunnel: w463 -> [w476 _]
              tunnel: w462 -> [w474 _]
              tunnel: w459 -> [w465 _]
              tunnel: [w466 _] -> w461
              frame False {
                n128 = call "_Compare Two Paths - Scalar.vi"("path2"=w465, "path1"=w474) -> ("relative path from 1 to 2"=w477:path)  [unwired: 1 in, 2 out]
                n129 = Build Path(base path=w476, name or relative path=w477) -> (appended path=w475:path)
                n130 = call <vilib>:"Check if File or Folder Exists.vi"("path"=w475) -> ("error out"=w471:errorcluster, "file or folder exists?"=w472:bool, "dup path"=w473:path)  [unwired: 8 in]
                n131 = case shown="True" w472 {
                  tunnel: w473 -> [w479 w483]
                  tunnel: [w479 w482] -> w470
                  tunnel: w471 -> [w478 w481]
                  tunnel: [w478 w480] -> w468
                  frame False {
                  }
                  frame True {
                    n132 = Delete(path (use dialog)=w483, error in=w481) -> (deleted path=w482:path, error out=w480:errorcluster)  [unwired: 3 in, 1 out]
                  }
                }
                n133 = Strip Path(path=w470) -> (stripped path=w469:path)  [unwired: 1 out]
                n134 = call <vilib>:"Create Directory Recursive.vi"("error in (no error)"=w468, "directory"=w469) -> ("error out"=w467:errorcluster)  [unwired: 3 in, 2 out]
                n135 = Move(source path=w465, error in=w467, 9:TRUE ("overwrite (F)"), 10:w470) -> (error out=w466:errorcluster)  [unwired: 1 in, 2 out]
              }
              frame True {
              }
            }
          }
          frame False {
            n136 = Empty String/Path?(string/path=w484) -> (empty?=w485:bool)
            n137 = case shown="False" w485 {
              tunnel: w488 -> [_ _]
              tunnel: w487 -> [_ _]
              tunnel: w484 -> [w490 _]
              tunnel: [w489 _] -> w486
              frame False {
                n138 = Delete(path (use dialog)=w490) -> (error out=w489:errorcluster)  [unwired: 4 in, 2 out]
              }
              frame True {
              }
            }
          }
        }
        n139 = call "Filter 1D Array_nevstop.vim"("items to filter"=w447, "array"=w448) -> ("filtered array"=w446:path[])  [unwired: 4 in, 1 out]
        n140 = Bundle By Name(cluster=w456, "Upload List"=w446, "Temp:UploadingFile"=path "") -> (w450:T6)
      }
      frame "FileSyncRountine: Remove Empty Container Folder" {
        n141 = Unbundle By Name(w496) -> ("Configuration.MonitoringFolder"=w495:path)  [unwired: 1 out]
        n142 = String To Path(string=w494) -> (path=w493:path)
        n143 = Empty String/Path?(string/path=w493) -> (empty?=w492:bool)
        n144 = case shown="False" w492 {
          tunnel: w498 -> [w504 w526]
          tunnel: [w503 w526] -> w497
          tunnel: w495 -> [w502 _]
          tunnel: w493 -> [w501 _]
          frame False {
            n145 = while {
              tunnel: w502 -> [w511]
              shift-right: [w507] -> w503
              shift-left: w504 -> [w508]
              shift-right: [w506] -> _
              shift-left: w501 -> [w512]
              stop <- w505 stop-if-true
              n146 = Strip Path(path=w512) -> (stripped path=w506:path)  [unwired: 1 out]
              n147 = List Folder(path=w506, error in=w508) -> (path out=w513:path, filenames=w519:string[], folder names=w518:string[], error out=w510:errorcluster)  [unwired: 2 in]
              n148 = Empty Array?(array=w519) -> (empty?=w517:bool)
              n149 = Empty Array?(array=w518) -> (empty?=w516:bool)
              n150 = Not Equal?(x=w511, y=w506) -> (x != y?=w514:bool)
              n151 = And(x=w517, y=w516) -> (x .and. y?=w515:bool)
              n152 = And(x=w514, y=w515) -> (x .and. y?=w509:bool)
              n153 = case shown="False" w509 {
                tunnel: w513 -> [_ w525]
                tunnel: w510 -> [w521 w524]
                tunnel: [w521 w523] -> w507
                tunnel: [TRUE FALSE] -> w505
                frame False {
                }
                frame True {
                  n154 = Delete(path (use dialog)=w525, error in=w524) -> (error out=w523:errorcluster)  [unwired: 3 in, 2 out]
                }
              }
            }
          }
          frame True {
          }
        }
      }
    }
  }
  "error out" <- w10
